vi "vPage_9234x1_CHx4.vi"() -> ()   [LabVIEW 2022 SP3]
uses:
  <vilib>/Utility/sysdir.llb/System Directory Type.ctl
  <vilib>/express/express analysis/Spectral/Block/exnSpectralBlock spectral measurements peak poly.vi
  <vilib>/express/express analysis/Spectral/Block/exnSpectralBlock spectral measurements peak DDT.vi
  <vilib>/express/express analysis/Spectral/XNode/ExpressSpectralMeasurementsBlockNode.xnode
panel:
  out "C1":i32
  in  "Show_FFT":bool
  in  "Show":bool
  in  "¸ê®Æ§¨\nµù°O>":string
  in  "Filter(Hz)\nLow-Cut":dbl=10.0
  out "DAQ Stoped":bool
  in  "SW \n(C1)":bool[](array[boolean])=[TRUE, TRUE, TRUE, TRUE, TRUE, TRUE, TRUE, TRUE]
  in  "Sample \nto Read":i32=25600
  in  "Sample\nRate":dbl=25600.0
  in  "Enable Saving":bool
  in  "Stop":bool
  out "C1-Save":bool
  out "C1-Trigger":bool
  out "C1-All":dynamicdata(graph)
  out "Statistics":T1(graph)
  out "C1-0":dynamicdata(graph)
  out "C1-2":dynamicdata(graph)
  out "C1-1":dynamicdata(graph)
  out "C1-3":dynamicdata(graph)
  # "使用前請先確認 \nDAQ 擷取卡設定"
  # "本頁畫面顯示為 觸發後訊號"
  # "FFT Filter by useing High-pass with Lower Cut-Off (Hz)"
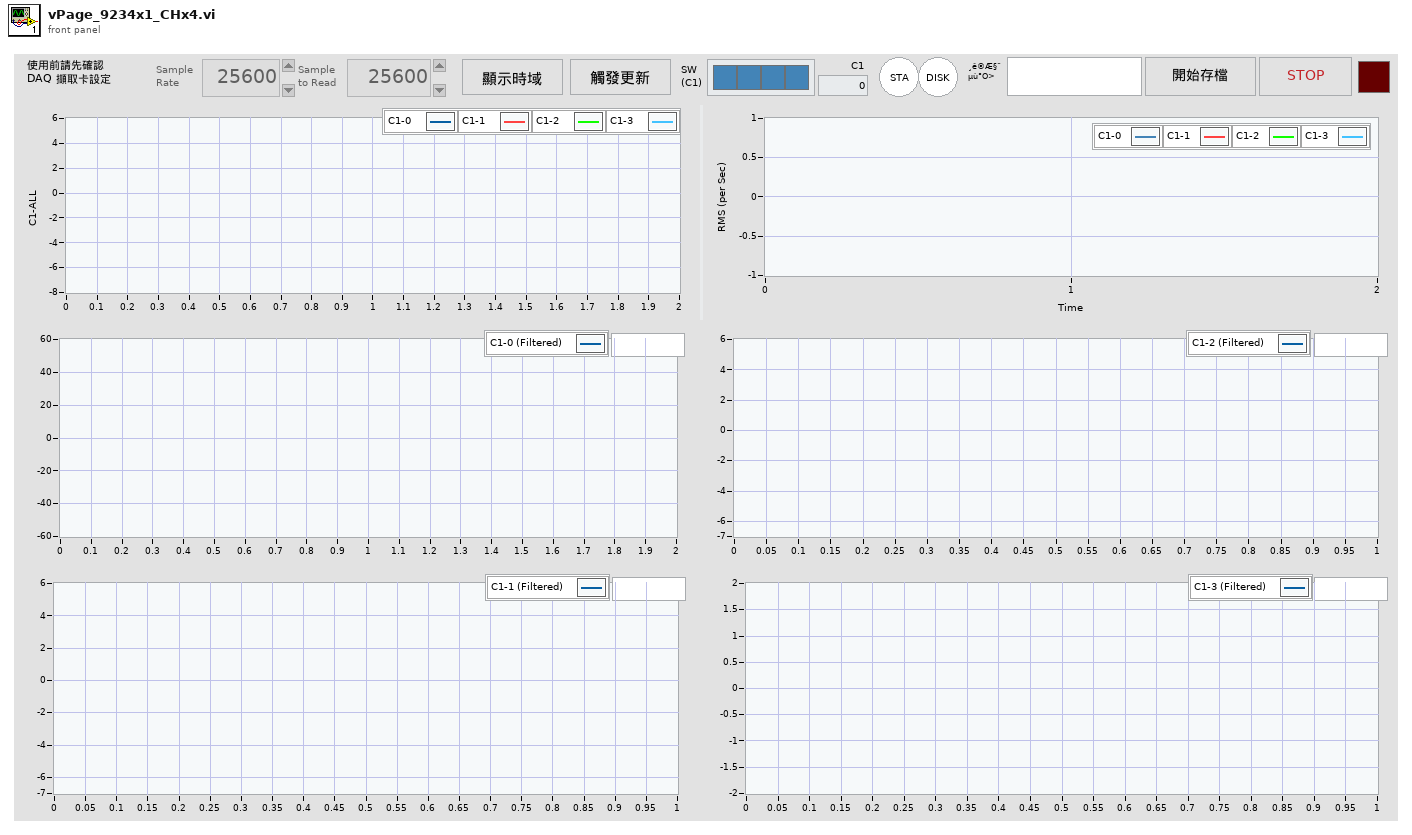
[diagram p1: front panel]
types:
  T1 = cluster{"Array[0]":dbl, "Array[1]":dbl, "Array[2]":dbl, "Array[3]":dbl}
  T2 = enum8{"Enabled", "Disabled", "Disabled and Grayed Out"}
  T3 = typedef "System Directory Type.ctl" = i32
  T4 = cluster{"task out":refnum<k21>, "data":dynamicdata}
  T5 = cluster{"averaging mode":u16, "weighting mode":u16, "number of averages":u32}
  T6 = cluster{"dB On (F)":bool, "unwrap phase (F)":bool, "convert to degree (F)":bool}
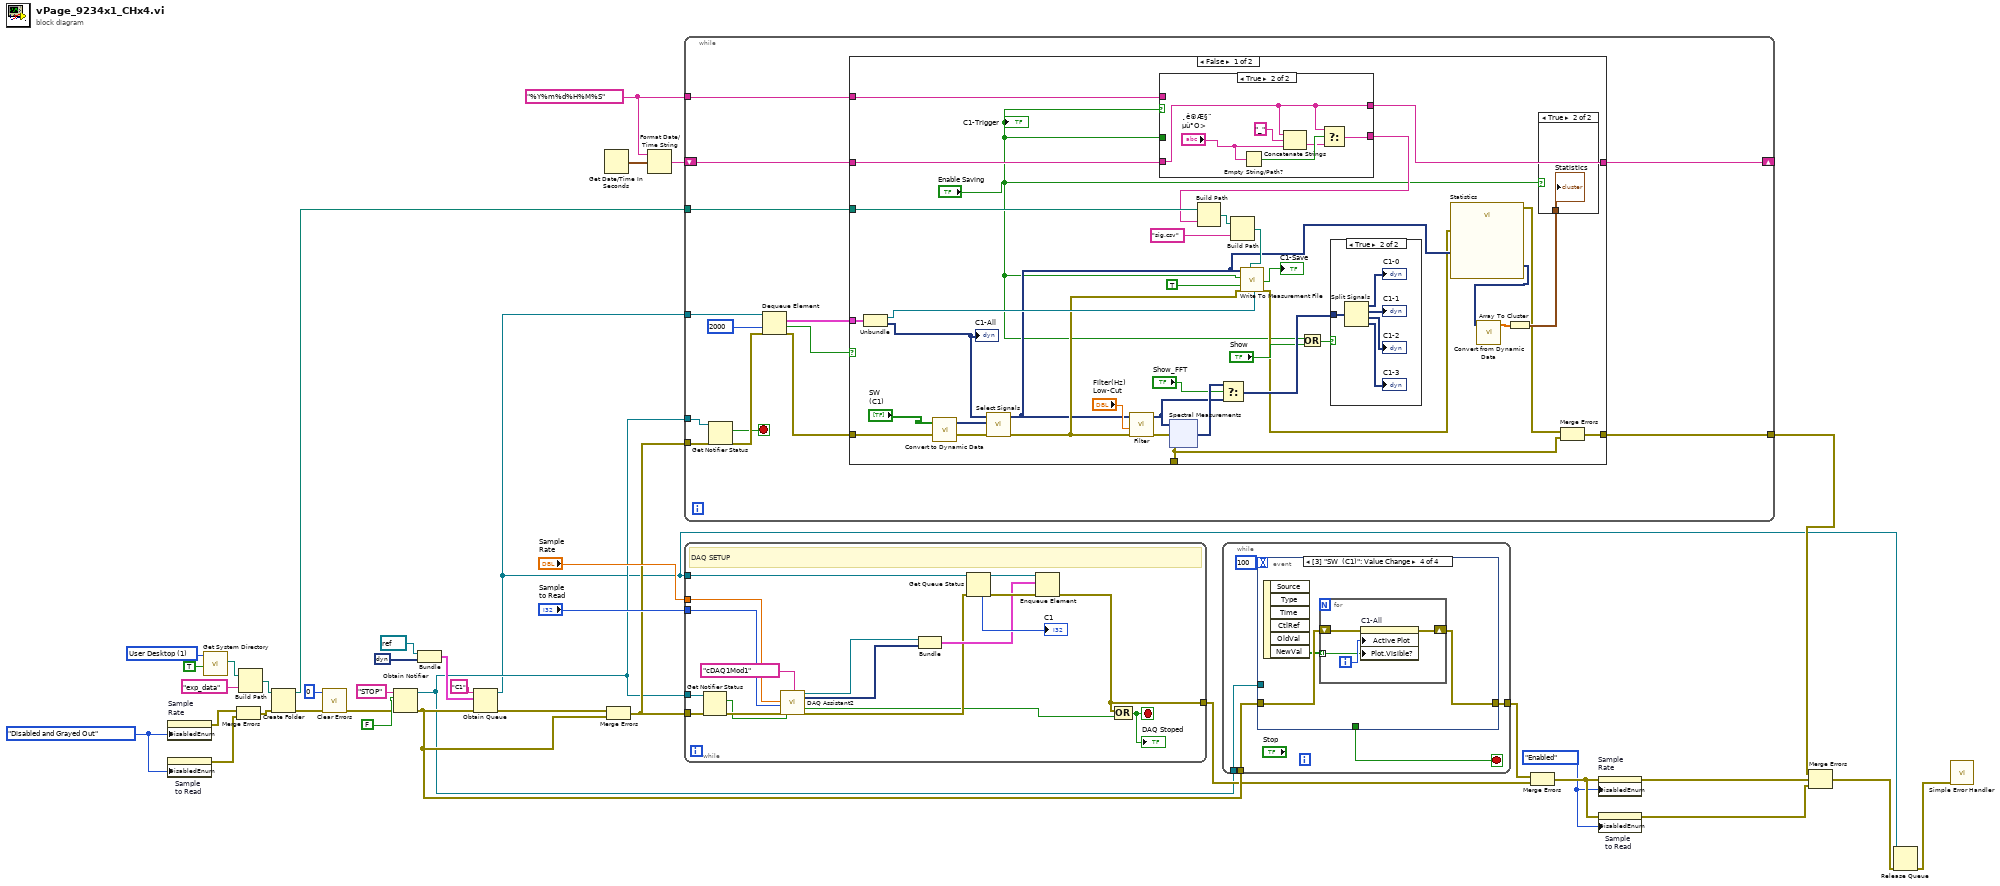
[diagram p0: block diagram]
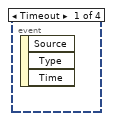
[diagram p2: hidden frame]
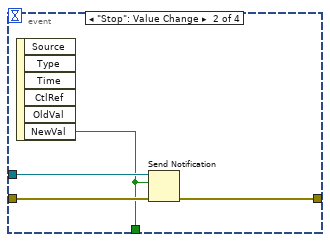
[diagram p3: hidden frame]
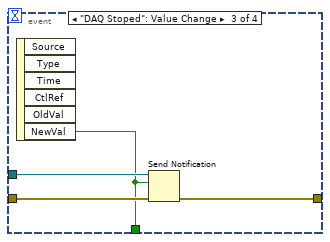
[diagram p4: hidden frame]
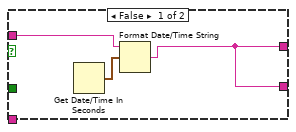
[diagram p7: hidden frame]
diagram:
  w7 = T2."Enabled" ("Disabled")
  w12 = T2."Disabled and Grayed Out" ("Disabled")
  w13 = "%Y%m%d%H%M%S" ("time format string (%c)")
  w23 = T3 1 items=["User Home"=0, "User Desktop"=1, "User Documents"=2, "User Application Data"=3, "User Preferences"=4, "User Temporary"=5, "Public Documents"=6, "Public Application Data"=7, "Public Preferences"=8, "Public Cache"=13, "System Core Libraries"=9, "System Installed Libraries"=10, "Application Files"=11, "Boot Volume Root"=12] ("system directory type")
  n1 = property on="Sample\nRate" class="DigNum (strict)"("DisabledEnum"=w12) -> (error out=w11:errorcluster)  [unwired: 2 in, 1 out]
  n2 = property on="Sample \nto Read" class="DigNum (strict)"("DisabledEnum"=w12) -> (error out=w9:errorcluster)  [unwired: 2 in, 1 out]
  n3 = call <vilib>:"Get System Directory.vi"("create directory if not found? (F)"=TRUE, "system directory type"=w23) -> ("system directory"=w25:path)  [unwired: 9 in]
  n4 = Merge Errors(w11, w9) -> (w10:errorcluster)
  n5 = Build Path(base path=w25, name or relative path="exp_data") -> (appended path=w19:path)
  n6 = Create Folder(path (use dialog)=w19, error in=w10) -> (created path=w18:path, error out=w21:errorcluster)  [unwired: 1 in, 1 out]
  n7 = call <vilib>:"Clear Errors.vi"("error in (no error)"=w21, "specific error code to clear (0: all)"=0) -> ("error out"=w20:errorcluster)  [unwired: 4 in, 1 out]
  n8 = Obtain Notifier(name (unnamed)="STOP", notification data type=FALSE, error in (no error)=w20) -> (notifier out=w14:refnum<notifier>, error out=w17:errorcluster)  [unwired: 1 in, 1 out]
  n9 = Bundle("task out"=refnum<k21> refnum, "data"=dynamicdata []) -> (w30:T4)  [unwired: 1 in]
  n10 = Obtain Queue(name (unnamed)="C1", element data type=w30, error in (no error)=w17) -> (queue out=w1:refnum<queue>, error out=w38:errorcluster)  [unwired: 2 in, 1 out]
  n11 = Get Date/Time In Seconds() -> (seconds since 1Jan1904=w28:timestamp)
  n12 = Merge Errors(w38, w17) -> (w29:errorcluster)
  n13 = Format Date/Time String(time format string (%c)=w13, seconds (now)=w28) -> (date/time string=w27:string)  [unwired: 1 in]
  n14 = while {
    tunnel: w29 -> [w52]
    tunnel: w14 -> [w50]
    tunnel: w1 -> [w49]
    shift-right: [w39] -> _
    shift-left: w27 -> [w43]
    tunnel: w18 -> [w44]
    tunnel: [w40] -> w2
    tunnel: w13 -> [w42]
    stop <- w47 stop-if-true
    n15 = Get Notifier Status(notifier=w50, error in (no error)=w52) -> (current notification=w47:bool, error out=w51:errorcluster)  [unwired: 3 out]
    n16 = Dequeue Element(queue=w49, timeout in ms (-1)=2000, error in (no error)=w51) -> (element=w45:T4, timed out?=w46:bool, error out=w41:errorcluster)  [unwired: 1 out]
    n17 = case shown="False" w46 {
      tunnel: w45 -> [w84 _]
      tunnel: w41 -> [w83 w112]
      tunnel: [w74 _] -> _
      tunnel: w43 -> [w80 w113]
      tunnel: [w79 w113] -> w39
      tunnel: w44 -> [w78 _]
      tunnel: [w73 w112] -> w40
      tunnel: w42 -> [w66 _]
      frame False {
        n18 = Unbundle(w84) -> ("task out"=w82:refnum<k21>, "data"=w62:dynamicdata)
        "C1-All" <- w62
        n19 = call "Convert to Dynamic Data"("Array"="SW \n(C1)") -> ("Dynamic Data Type"=w70:dynamicdata)  [unwired: 3 in]
        n20 = call "Select Signals"("error in (no error)"=w83, "Selector Input"=w70, "Signals"=w62) -> ("error out"=w81:errorcluster, "Signal Out"=w59:dynamicdata)  [unwired: 7 in]
        n21 = call "Filter"("error in (no error)"=w81, "Lower Cut-Off"="Filter(Hz)\nLow-Cut", "Signal"=w59) -> ("error out"=w86:errorcluster, "Filtered Signal"=w71:dynamicdata)  [unwired: 7 in]
        n22 = case shown="True" "Enable Saving" {
          tunnel: [w93 w97] -> w79
          tunnel: "Enable Saving" -> [_ _]
          tunnel: w80 -> [_ w97]
          tunnel: [w93 w99] -> w67
          tunnel: w66 -> [w94 _]
          frame False {
            n23 = Get Date/Time In Seconds() -> (seconds since 1Jan1904=w95:timestamp)
            n24 = Format Date/Time String(time format string (%c)=w94, seconds (now)=w95) -> (date/time string=w93:string)  [unwired: 1 in]
          }
          frame True {
            n25 = Empty String/Path?(string/path="¸ê®Æ§¨\nµù°O>") -> (empty?=w101:bool)
            n26 = Concatenate Strings(w97, "_" ("string"), "¸ê®Æ§¨\nµù°O>") -> (w100:string)
            n27 = Select(t=w97, s=w101, f=w100) -> (s? t:f=w99:string)
          }
        }
        n28 = xnode ("Spectral Measurements")("Signals"=w71, "error in (no error)"=w86) -> ("FFT - (Peak)"=w72:dynamicdata, "error out"=w74:errorcluster)  [unwired: 1 out]
        n29 = Build Path(base path=w78, name or relative path=w67) -> (appended path=w77:path)
        n30 = Select(t=w72, s="Show_FFT", f=w71) -> (s? t:f=w69:dynamicdata)
        n31 = Build Path(base path=w77, name or relative path="sig.csv") -> (appended path=w75:path)
        n32 = call "Write To Measurement File"("Signals"=w59, "Enable"="Enable Saving", "new_file"=TRUE, "error in (no error)"=w81, "Filename"=w75, "DAQmx Task"=w82) -> ("Saving Data"=→"C1-Save":bool, "error out"=w55:errorcluster)  [unwired: 11 in, 1 out]
        n33 = Or(x="Enable Saving", y="Show") -> (x .or. y?=w65:bool)
        n34 = case shown="True" w65 {
          tunnel: w69 -> [_ w89]
          frame False {
          }
          frame True {
            n35 = Split Signals(w89) -> (→"C1-0":dynamicdata, →"C1-1":dynamicdata, →"C1-2":dynamicdata, →"C1-3":dynamicdata)  [unwired: 4 in]
          }
        }
        n36 = call "Statistics"("Signals"=w59, "error in (no error)"=w55) -> ("RMS"=w58:dynamicdata, "error out"=w54:errorcluster)  [unwired: 24 in]
        n37 = call "Convert from Dynamic Data"("Dynamic Data Type"=w58) -> ("Array"=w57:dbl[])  [unwired: 3 in]
        n38 = Array To Cluster(array=w57) -> (cluster=w56:T1)
        n39 = case shown="True" "Enable Saving" {
          tunnel: w56 -> [_ w87]
          frame False {
          }
          frame True {
            "Statistics" <- w87
          }
        }
        n40 = Merge Errors(w54, w74) -> (w73:errorcluster)
        "C1-Trigger" <- "Enable Saving"
      }
      frame True {
      }
    }
  }
  n41 = while {
    tunnel: [w130] -> w15
    tunnel: w1 -> [w127]
    tunnel: w29 -> [w126]
    tunnel: w14 -> [w125]
    tunnel: "Sample \nto Read" -> [w119]
    tunnel: "Sample\nRate" -> [w120]
    stop <- w128 stop-if-true
    # "DAQ SETUP"
    n42 = Get Notifier Status(notifier=w125, error in (no error)=w126) -> (current notification=w118:bool, error out=w122:errorcluster)  [unwired: 3 out]
    n43 = call "DAQ Assistant2"("rate"=w120, "number of samples"=w119, "error in"=w122, "stop (F)"=w118, "device name"=tag "cDAQ1Mod1") -> ("task out"=w116:refnum<k21>, "data"=w115:dynamicdata, "stopped"=w117:bool, "error out"=w121:errorcluster)  [unwired: 11 in]
    n44 = Bundle("task out"=w116, "data"=w115) -> (w123:T4)  [unwired: 1 in]
    n45 = Get Queue Status(queue=w127, error in (no error)=w121) -> (queue out=w124:refnum<queue>, error out=w131:errorcluster, # elements in queue=→"C1":i32)  [unwired: 1 in, 5 out]
    n46 = Enqueue Element(queue=w124, element=w123, error in (no error)=w131) -> (error out=w130:errorcluster)  [unwired: 1 in, 2 out]
    n47 = Compound Arithmetic op=OR(w130, w117) -> (w128:bool)
    "DAQ Stoped" <- w128
  }
  n48 = while {
    tunnel: w17 -> [w136]
    tunnel: [w135] -> w16
    tunnel: w14 -> [w134]
    stop <- w133 stop-if-true
    n49 = event shown="[3] \"SW  (C1)\": Value Change" {
      selector: _ -> [_ _ _ _]
      dyn-events: _ -> [_ _ _ _]
      timeout: 100 -> [_ _ _ _]
      tunnel: w136 -> [_ w140 w144 w147]
      tunnel: [_ w139 w143 w146] -> w135
      tunnel: w134 -> [_ w138 w142 _]
      tunnel: [_ w137 w141 _] -> w133
      event Timeout {
        n50 = event-data() -> ()  [unwired: 1 in, 3 out]
      }
      event "Stop": Value Change {
        n51 = event-data() -> ("NewVal"=w137:bool)  [unwired: 1 in, 5 out]
        n52 = Send Notification(notification=w137, notifier=w138, error in (no error)=w140) -> (error out=w139:errorcluster)  [unwired: 1 out]
      }
      event "DAQ Stoped": Value Change {
        n53 = event-data() -> ("NewVal"=w141:bool)  [unwired: 1 in, 5 out]
        n54 = Send Notification(notification=w141, notifier=w142, error in (no error)=w144) -> (error out=w143:errorcluster)  [unwired: 1 out]
      }
      event "SW \n(C1)": Value Change {
        n55 = event-data() -> ("NewVal"=w145:bool[])  [unwired: 1 in, 5 out]
        n56 = for {
          shift-right: [w148] -> w146
          shift-left: w147 -> [w150]
          tunnel: w145 -> [w149] mode=indexing
          i -> [w151]
          n57 = property on="C1-All" class="WFGraph (strict)"(error in=w150, "Active Plot"=w151, "Plot.Visible?"=w149) -> (error out=w148:errorcluster)  [unwired: 1 in, 1 out]
        }
      }
    }
  }
  n58 = Merge Errors(w16, w15) -> (w8:errorcluster)
  n59 = property on="Sample\nRate" class="DigNum (strict)"(error in=w8, "DisabledEnum"=w7) -> (error out=w6:errorcluster)  [unwired: 1 in, 1 out]
  n60 = property on="Sample \nto Read" class="DigNum (strict)"(error in=w8, "DisabledEnum"=w7) -> (error out=w5:errorcluster)  [unwired: 1 in, 1 out]
  n61 = Merge Errors(w2, w6, w5) -> (w3:errorcluster)
  n62 = Release Queue(queue=w1, error in (no error)=w3) -> (error out=w4:errorcluster)  [unwired: 1 in, 2 out]
  n63 = call <vilib>:"Simple Error Handler.vi"("error in (no error)"=w4) -> ()  [unwired: 4 in, 5 out]
